vi "Read Color.vi"(9 "Pane in":refnum<class "Pane.lvclass">) -> (3 "Pane out":refnum<class "Pane.lvclass">, 4 "Color":u32(colorbox))   [LabVIEW 2014, in "Raspberry Pi Compatible Compiler for LabVIEW.lvlib" / "Pane.lvclass"]
uses:
  Pane.lvclass
  Pane.lvclass/Pane.ctl
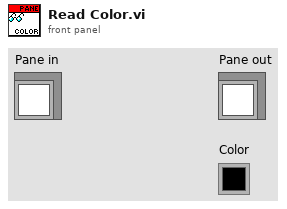
[diagram p1: front panel]
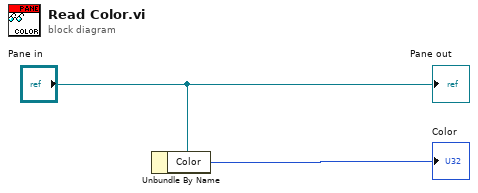
[diagram p0: block diagram]
diagram:
  n1 = Unbundle By Name("Pane in") -> ("Color"=→"Color":u32)
  "Pane out" <- "Pane in"
